vi "E710_Initialisation.vi"(5 "error IO":errorcluster) -> (14 "Position":dbl[](array[numeric]) format="%.6f", 15 "ATZ successful?":bool[](array[boolean]), 16 "Conn. Axes":string[](array[string]), 17 "Identification":string, 19 "error out":errorcluster)   [LabVIEW 2013]
uses:
  Utilities/controls/ctlSeqFNs_PI_SysNr.ctl
  Variables/GlobalSetGetPositionParameters.vi
  Variables/GlobalSetConfigurationPhysikalInstruments.vi
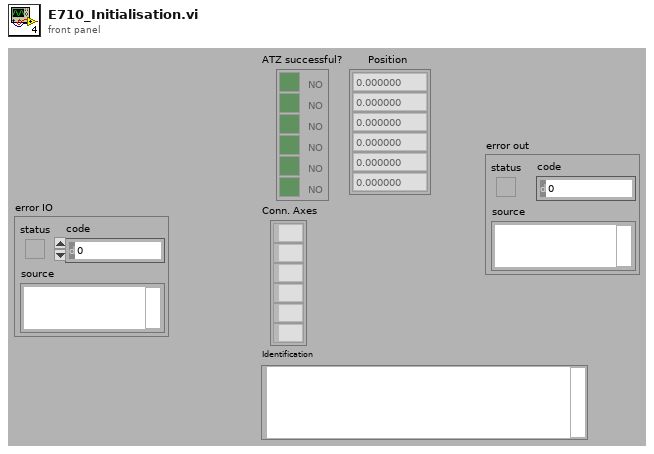
[diagram p1: front panel]
types:
  T1 = typedef "ctlSeqFNs_PI_SysNr.ctl" = enum16{"Zero", "E517", "E710"}
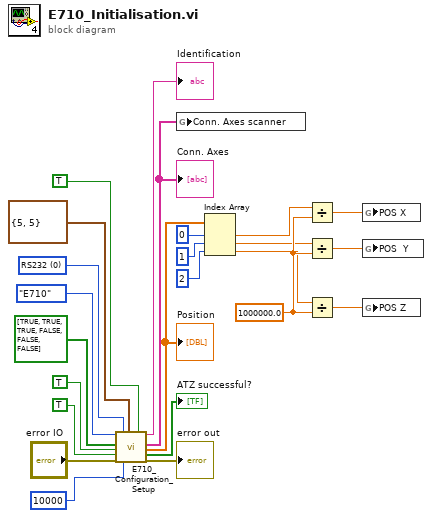
[diagram p0: block diagram]
diagram:
  w12 = 1000000.0 ("y")
  w24 = u16 0 items=["RS232", "GPIB"] ("Interface")
  n1 = call "E710_Configuration_Setup.vi"("System no."=ctlSeqFNs_PI_SysNr."E710" ("STATE"), "Are stages connected?"=bool[] [TRUE, TRUE, TRUE, FALSE, FALSE, FALSE], "Change servo \nstatus to ON?"=TRUE ("Change servo \nstatus to ON?"), "Perform autozero?"=TRUE, "error in"="error IO", "Interface"=w24, "Timeout"=u32 10000, "RS232 settings"=cluster{"Portnumber":i32, "Baudrate":u16} {"Portnumber"=5, "Baudrate"=5}, "Move to middle?"=TRUE) -> ("Identification"=→"Identification":string, "Conn. Axes"=w3:string[], "Position"=w19:dbl[], "ATZ successful?"=→"ATZ successful?":bool[], "error out"=→"error out":errorcluster)  [unwired: 6 in]
  "Position" <- w19
  "Conn. Axes" <- w3
  n2 = global write "GlobalSetConfigurationPhysikalInstruments.vi" "Conn. Axes scanner"(w3) -> ()
  n3 = Index Array(array=w19, index #1=0 ("index"), index #2=1 ("index"), index #3=2 ("index")) -> (element #1=w9:dbl, element #2=w10:dbl, element #3=w11:dbl)
  n4 = Divide(x=w9, y=w12) -> (x/y=w14:dbl)
  n5 = Divide(x=w10, y=w12) -> (x/y=w15:dbl)
  n6 = Divide(x=w11, y=w12) -> (x/y=w13:dbl)
  n7 = global write "GlobalSetGetPositionParameters.vi" "POS X"(w14) -> ()
  n8 = global write "GlobalSetGetPositionParameters.vi" "POS  Y"(w15) -> ()
  n9 = global write "GlobalSetGetPositionParameters.vi" "POS Z"(w13) -> ()
